vi "Trigger Detector (XY).vi"(0 "data in":T4(array[cluster]), 1 "reset? (F)":bool, 5 "triggers definition":T3(array[cluster]), 11 "error in (no error)":errorcluster) -> (4 "triggers":T2(array[cluster]), 6 "actual trigger state":T1[](array[typedef]), 15 "error out":errorcluster)   [LabVIEW 2014, in "NI_EP_Power Quality.lvlib"]
doc: "Detects crossing of limits for the measurement that you specify and returns triggers if occur.\n\nThis VI supports measuring single-line and multiple-line systems except the DBL instance. Use the DBL instance to measure one channel on one line at one time."
uses:
  <vilib>/addons/Electrical Power/PQ/NI_EP_Power Quality.lvlib
  <vilib>/addons/Electrical Power/PQ/Common/Controls/ep_Trigger State.ctl
  <vilib>/addons/Electrical Power/PQ/Triggers/subVIs/ep_Trigger Definition.ctl
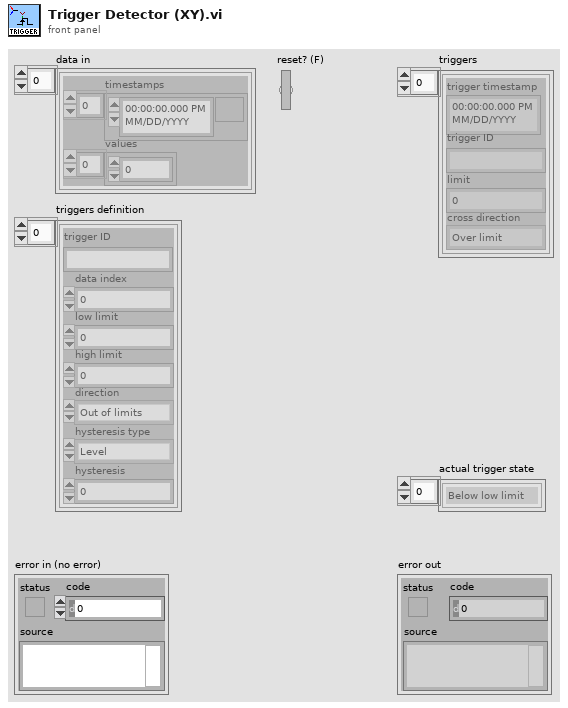
[diagram p1: front panel]
types:
  T1 = typedef "NI_EP_Power Quality.lvlib/ep_Trigger State.ctl" = enum16{"Below low limit", "In the limits", "Over high limit"}
  T2 = cluster{"trigger timestamp":timestamp, "trigger ID":string, "limit":dbl, "cross direction":enum16{"Over limit", "Below limit"}}[]
  T3 = cluster{"trigger ID":string, "data index":u32, "low limit":dbl, "high limit":dbl, "direction":enum16{"Out of limits", "Back to limits", "Both"}, "hysteresis type":enum16{"Level", "Time"}, "hysteresis":dbl}[]
  T4 = cluster{"timestamps":timestamp[], "values":dbl[]}[]
  T5 = cluster{"trigger time":timestamp, "trigger unique id":string, "limit":dbl, "cross direction":enum16{"Over limit", "Below limit"}}[]
  T6 = typedef "NI_EP_Power Quality.lvlib/ep_Trigger Definition.ctl" = cluster{"trigger ID":string, "low limit":dbl, "high limit":dbl, "direction":enum16{"Out of limits", "Back to limits", "Both"}, "hysteresis type":enum16{"Level", "Time"}, "hysteresis":dbl}
  T7 = cluster{"Lo in progr.":bool, "Lo in progr.":bool, timestamp, timestamp}[]
  T8 = enum16{"Out of limits", "Back to limits", "Both"}
  T9 = cluster{"timestamps":timestamp[], "values":dbl[]}
  T10 = cluster{"Lo in progr.":bool, "Lo in progr.":bool, timestamp, timestamp}
  T11 = cluster{"Lo in progr.":bool, "Hi in progr.":bool, "Lo trig. time":timestamp, "Hi trig. time":timestamp}
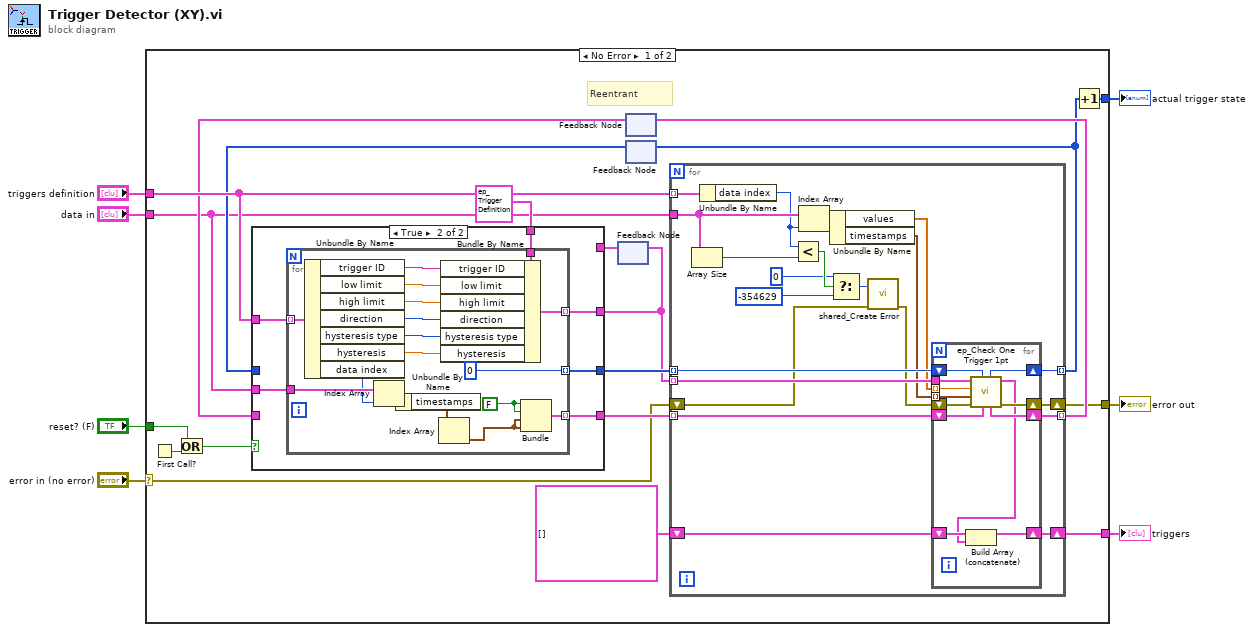
[diagram p0: block diagram]
diagram:
  n1 = case shown="No Error" "error in (no error)" {
    selector: "error in (no error)" -> [w10 w86]
    tunnel: "data in" -> [w11 _]
    tunnel: "reset? (F)" -> [w25 _]
    tunnel: "triggers definition" -> [w23 _]
    tunnel: [w13 _] -> w6
    tunnel: [w12 w86] -> w7
    tunnel: [w8 _] -> w1
    frame No Error {
      # "Reentrant"
      n2 = First Call?() -> (First Call?: T/F=w26:bool)
      n3 = Or(x=w25, y=w26) -> (x .or. y?=w24:bool)
      n4 = feedback #1() -> (w16:T6[])  [unwired: 1 in]
      n5 = feedback #2() -> (w17:T7)  [unwired: 1 in]
      n6 = feedback #3() -> (w19:i8[])  [unwired: 1 in]
      n7 = case shown="True" w24 {
        tunnel: w23 -> [_ w35]
        tunnel: [w27 w34] -> w15
        tunnel: T6 {"trigger ID"="", "low limit"=0.0, "high limit"=0.0, "direction"=enum."Out of limits", "hysteresis type"=enum."Level", "hysteresis"=0.0} ("trigger definition") -> [_ w33]
        tunnel: [w29 w32] -> w21
        tunnel: [w28 w31] -> w20
        tunnel: w19 -> [w28 _]
        tunnel: w17 -> [w29 _]
        tunnel: w16 -> [w27 _]
        tunnel: w11 -> [_ w30]
        frame False {
        }
        frame True {
          n8 = for {
            tunnel: w35 -> [w48] mode=indexing
            tunnel: [w47] -> w34 mode=indexing
            tunnel: w33 -> [w46]
            tunnel: [w43] -> w32 mode=indexing
            tunnel: [i8 0] -> w31 mode=indexing
            tunnel: w30 -> [w40]
            w44 = FALSE ("Lo in progr.")
            n9 = Unbundle By Name(w48) -> ("trigger ID"=w51:string, "low limit"=w42:dbl, "high limit"=w41:dbl, "direction"=w50:T8, "hysteresis type"=w49:enum16{"Level", "Time"}, "hysteresis"=w52:dbl, "data index"=w39:u32)
            n10 = Index Array(array=w40, index=w39) -> (element=w38:T9)
            n11 = Unbundle By Name(w38) -> ("timestamps"=w37:timestamp[])
            n12 = Index Array(array=w37) -> (element=w36:timestamp)  [unwired: 1 in]
            n13 = Bundle By Name(cluster=w46, "trigger ID"=w51, "low limit"=w42, "high limit"=w41, "direction"=w50, "hysteresis type"=w49, "hysteresis"=w52) -> (w47:T6)
            n14 = Bundle("Lo in progr."=w44, "Lo in progr."=w44, w36, w36) -> (w43:T10)  [unwired: 1 in]
          }
        }
      }
      n15 = feedback-in #1(w15) -> ()
      n16 = for {
        tunnel: w23 -> [w69] mode=indexing
        tunnel: w11 -> [w66]
        tunnel: w21 -> [w68] mode=indexing
        tunnel: w20 -> [w72] mode=indexing
        tunnel: [w71] -> w9 mode=indexing
        tunnel: [w70] -> w18 mode=indexing
        tunnel: w15 -> [w73] mode=indexing
        shift-right: [w60] -> w13
        shift-left: T5 [] -> [w61]
        shift-right: [w67] -> w12
        shift-left: w10 -> [w54]
        n17 = Array Size(array=w66) -> (size(s)=w64:i32)
        n18 = Unbundle By Name(w69) -> ("data index"=w65:u32)
        n19 = Less?(x=w65, y=w64) -> (x < y?=w63:bool)
        n20 = Index Array(array=w66, index=w65) -> (element=w62:T9)
        n21 = Unbundle By Name(w62) -> ("values"=w59:dbl[], "timestamps"=w58:timestamp[])
        n22 = Select(t=0 ("error code (0)"), s=w63, f=-354629 ("error code (0)")) -> (s? t:f=w55:i32)
        n23 = call <vilib>:"shared_Create Error.vi"("error in (no error)"=w54, "error code (0)"=w55) -> ("error out"=w53:errorcluster)  [unwired: 9 in]
        n24 = for {
          tunnel: w73 -> [w85]
          tunnel: w58 -> [w82] mode=indexing
          shift-right: [w83] -> w71
          shift-left: w72 -> [w84]
          shift-right: [w79] -> w67
          shift-left: w53 -> [w78]
          shift-right: [w81] -> w70
          shift-left: w68 -> [w80]
          shift-right: [w75] -> w60
          shift-left: w61 -> [w77]
          tunnel: w59 -> [w74] mode=indexing
          n25 = call <vilib>:"ep_Check One Trigger 1pt.vi"("trig. local in"=w80, "prev. state in"=w84, "error in (no error)"=w78, "data time stamp"=w82, "value in"=w74, "trigger definition"=w85) -> ("error out"=w79:errorcluster, "triggers list"=w76:T5, "trig. local out"=w81:T11, "state out"=w83:i8)  [unwired: 2 in]
          n26 = Build Array (concatenate)(w77, w76) -> (w75:T5)
        }
      }
      n27 = feedback-in #2(w18) -> ()
      n28 = feedback-in #3(w9) -> ()
      n29 = Increment(x=w9) -> (x+1=w8:i8[])
    }
    frame Error {
    }
  }
  "error out" <- w7
  "triggers" <- w6
  "actual trigger state" <- w1
